vi "AddLift.vi"(7 "ArrayHigh":u32[][](array[numeric]), 8 "Front":bool, 9 "Back":bool, 10 "ArrayLow":u32[][](array[numeric]), 11 "Refnum in":T1) -> (3 "Refnum out":T1)   [LabVIEW 2018]
uses:
  <vilib>/vision/Image Controls.llb/IMAQ Image.ctl
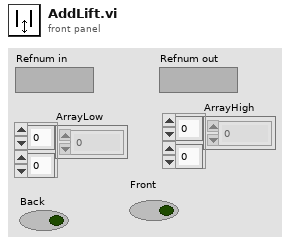
[diagram p1: front panel]
types:
  T1 = typedef "IMAQ Image.ctl" = refnum<image>
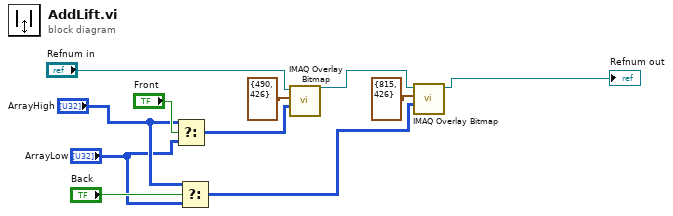
[diagram p0: block diagram]
diagram:
  n1 = Select(t="ArrayHigh", s="Front", f="ArrayLow") -> (s? t:f=w9:u32[][])
  n2 = Select(t="ArrayHigh", s="Back", f="ArrayLow") -> (s? t:f=w3:u32[][])
  n3 = call "IMAQ Overlay Bitmap"("Bitmap"=w9, "Top Left Point"=cluster{"X":i32, "Y":i32} {"X"=490, "Y"=426}, "Image"="Refnum in") -> ("Image Out"=w4:T1)  [unwired: 7 in, 1 out]
  n4 = call "IMAQ Overlay Bitmap"("Bitmap"=w3, "Top Left Point"=cluster{"X":i32, "Y":i32} {"X"=815, "Y"=426}, "Image"=w4) -> ("Image Out"=→"Refnum out":T1)  [unwired: 7 in, 1 out]
